vi "Read Source Channels.vi"(8 "error in (no error)":errorcluster, 11 "SLSC Switch Init Parameters in":refnum<class "SLSC Switch Init Parameters.lvclass">) -> (0 "error out":errorcluster, 2 "Source Channels":string[](array[string]), 3 "SLSC Switch Init Parameters out":refnum<class "SLSC Switch Init Parameters.lvclass">)   [LabVIEW 2020, in "SLSC Switch Messaging.lvlib" / "SLSC Switch Init Parameters.lvclass"]
uses:
  SLSC Switch Init Parameters.lvclass
  SLSC Switch Init Parameters.lvclass/SLSC Switch Init Parameters.ctl
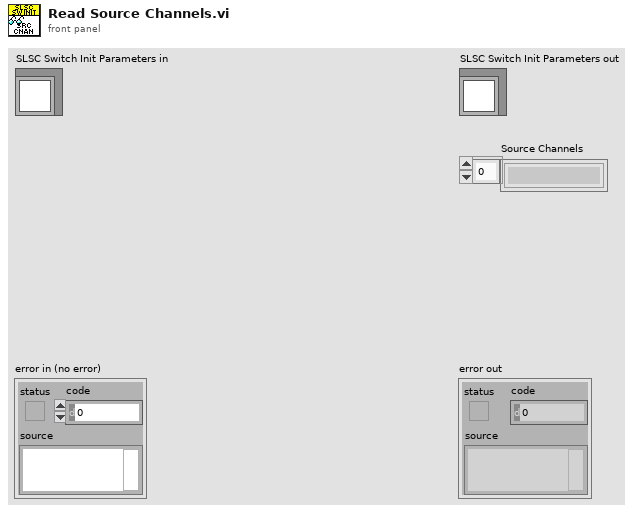
[diagram p1: front panel]
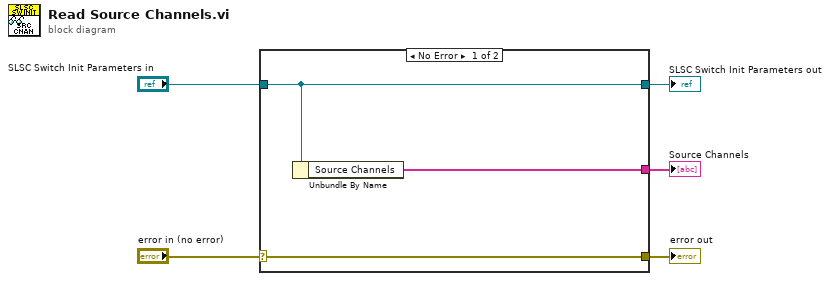
[diagram p0: block diagram]
diagram:
  n1 = case shown="No Error" "error in (no error)" {
    selector: "error in (no error)" -> [w8 w9]
    tunnel: [w8 w9] -> w4
    tunnel: [w7 w10] -> w2
    tunnel: "SLSC Switch Init Parameters in" -> [w7 w10]
    tunnel: [w6 _] -> w1
    frame No Error {
      n2 = Unbundle By Name(w7) -> ("Source Channels"=w6:string[])
    }
    frame Error {
    }
  }
  "error out" <- w4
  "SLSC Switch Init Parameters out" <- w2
  "Source Channels" <- w1
